vi "Alarm Limit Handler.vi"(8 "Min Limit":dbl, 11 "Max Limit":dbl) -> ()   [LabVIEW 2014]
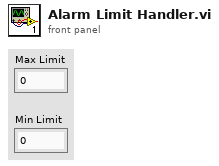
[diagram p1: front panel]
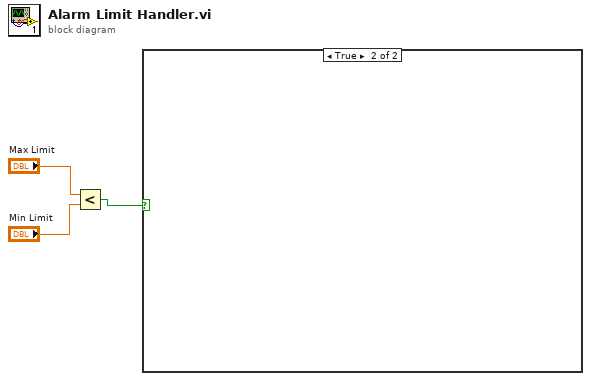
[diagram p0: block diagram]
diagram:
  n1 = Less?(x="Max Limit", y="Min Limit") -> (x < y?=w1:bool)
  n2 = case shown="True" w1 {
    frame False {
    }
    frame True {
    }
  }
